vi "compile_commands.vi"(6 "Zero Forces and Moment":bool, 7 "Zero Angle":bool, 9 "Zero Airspeed & Pressures":bool, 10 "Desired Airspeed (m/s)":dbl, 11 "Zero ELD Probe Location":bool) -> (3 "Array":dbl[](array[numeric]))   [LabVIEW 2019]
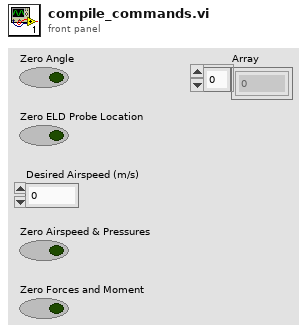
[diagram p1: front panel]
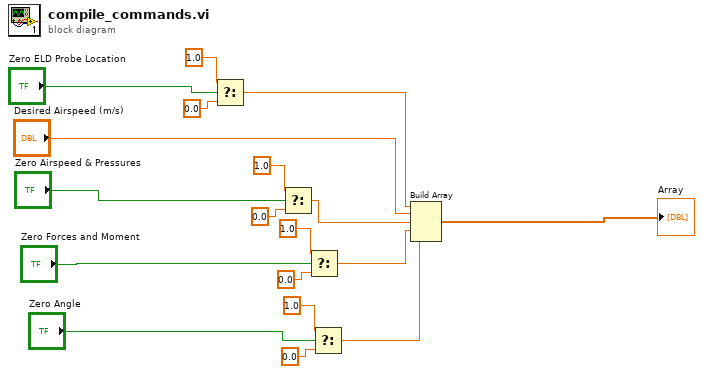
[diagram p0: block diagram]
diagram:
  n1 = Select(t=1.0, s="Zero ELD Probe Location", f=0.0) -> (s? t:f=w13:dbl)
  n2 = Select(t=1.0, s="Zero Airspeed & Pressures", f=0.0) -> (s? t:f=w15:dbl)
  n3 = Select(t=1.0, s="Zero Forces and Moment", f=0.0) -> (s? t:f=w16:dbl)
  n4 = Select(t=1.0, s="Zero Angle", f=0.0) -> (s? t:f=w17:dbl)
  n5 = Build Array(w13, "Desired Airspeed (m/s)", w15, w16, w17) -> (→"Array":dbl[])
